vi "UDPTeste.vi"(11 "UDP RX":T1={"Port:"=10020, "Server IP:"="224.5.23.2", "Local IP:"="224.5.23.2", "RX"=FALSE}) -> (2 "RX":bool, 3 "data camera":u8[](array[numeric]))   [LabVIEW 2018]
uses:
  Control/SSL UDP Address.ctl
  <vilib>/Utility/tcp.llb/UDP Multicast Read-Only Open.vi
panel:
  out "error out":errorcluster
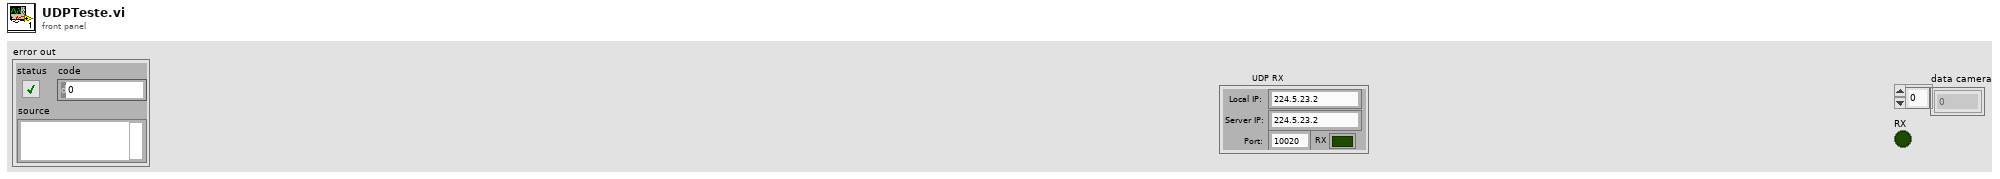
[diagram p1: front panel]
types:
  T1 = typedef "SSL UDP Address.ctl" = cluster{"Port:":u16, "Server IP:":string, "Local IP:":string, "RX":bool}
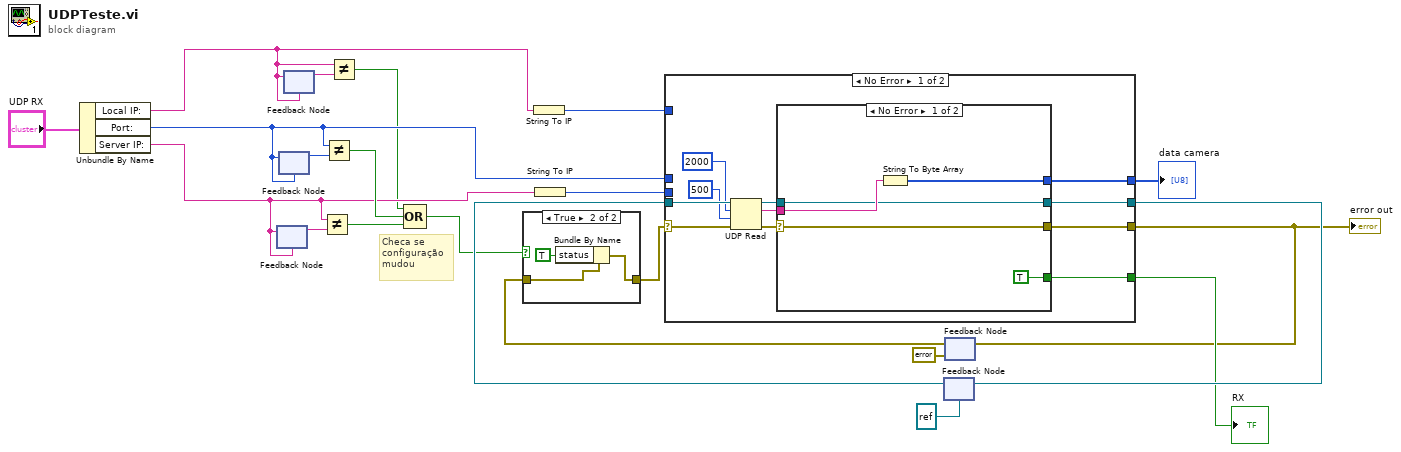
[diagram p0: block diagram]
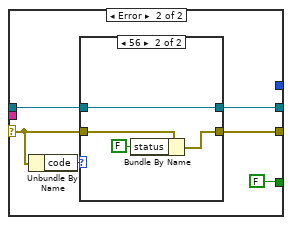
[diagram p3: hidden frame]
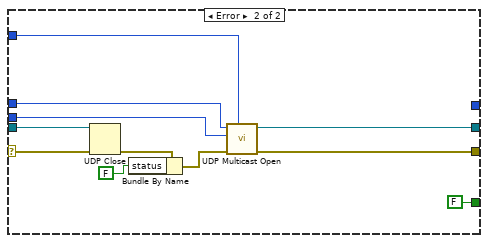
[diagram p5: hidden frame]
diagram:
  # "Checa se \nconfiguração\nmudou"
  n1 = Unbundle By Name("UDP RX") -> ("Local IP:"=w6:string, "Port:"=w10:u16, "Server IP:"=w9:string)
  n2 = feedback #1(w9) -> (w15:string)
  n3 = feedback-in #1(w9) -> ()
  n4 = feedback #2(w10) -> (w13:u16)
  n5 = feedback-in #2(w10) -> ()
  n6 = feedback #3(w6) -> (w8:string)
  n7 = feedback-in #3(w6) -> ()
  n8 = Not Equal?(x=w9, y=w15) -> (x != y?=w14:bool)
  n9 = Not Equal?(x=w10, y=w13) -> (x != y?=w12:bool)
  n10 = Not Equal?(x=w6, y=w8) -> (x != y?=w7:bool)
  n11 = Compound Arithmetic op=OR(w7, w12, w14) -> (w11:bool)
  n12 = String To IP(1:w6) -> (0:w5:u32)
  n13 = String To IP(1:w9) -> (0:w20:u32)
  n14 = feedback #4(refnum<k16> refnum ("connection ID")) -> (w21:refnum<k16>)
  n15 = feedback #5(errorcluster {"status"=TRUE, "code"=0, "source"=""} ("error out")) -> (w17:errorcluster)
  n16 = case shown="True" w11 {
    tunnel: w17 -> [w23 w25]
    tunnel: [w23 w24] -> w16
    frame False {
    }
    frame True {
      n17 = Bundle By Name(cluster=w25, "status"=TRUE) -> (w24:errorcluster)
    }
  }
  n18 = case shown="No Error" w16 {
    selector: w16 -> [w28 w56]
    tunnel: w21 -> [w37 w62]
    tunnel: [w36 w64] -> w3
    tunnel: [w35 w65] -> w22
    tunnel: w10 -> [_ w63]
    tunnel: w20 -> [_ w61]
    tunnel: [w29 FALSE] -> w4
    tunnel: w5 -> [_ w55]
    tunnel: [w27 _] -> w2
    frame No Error {
      n19 = UDP Read(connection ID=w37, max size (548)=2000, timeout ms (25000)=500, 8:w28) -> (data out=w32:string, error out=w30:errorcluster, 3:w31:refnum<k16>)  [unwired: 2 out]
      n20 = case shown="No Error" w30 {
        selector: w30 -> [w39 w43]
        tunnel: w32 -> [w42 _]
        tunnel: [w39 w45] -> w36
        tunnel: [w41 w46] -> w35
        tunnel: w31 -> [w41 w47]
        tunnel: [TRUE FALSE] -> w29
        tunnel: [w38 _] -> w27
        frame No Error {
          n21 = String To Byte Array(string=w42) -> (unsigned byte array=w38:u8[])
        }
        frame Error {
          n22 = Unbundle By Name(w43) -> ("code"=w48:i32)
          n23 = case shown="56" w48 {
            tunnel: w43 -> [w50 w54]
            tunnel: [w50 w52] -> w45
            tunnel: w47 -> [w49 w51]
            tunnel: [w49 w51] -> w46
            frame Default {
            }
            frame 56 {
              n24 = Bundle By Name(cluster=w54, "status"=FALSE) -> (w52:errorcluster)
            }
          }
        }
      }
    }
    frame Error {
      n25 = UDP Close(connection ID=w62, 8:w56) -> (error out=w59:errorcluster)  [unwired: 1 out]
      n26 = Bundle By Name(cluster=w59, "status"=FALSE) -> (w57:errorcluster)
      n27 = call-poly <vilib>:"UDP Multicast Open.vi"("net address"=w55, "error in (no error)"=w57, "multicast addr"=w61, "port"=w63) -> ("error out"=w64:errorcluster, "connection ID"=w65:refnum<k16>)  [unwired: 5 in, 1 out]
    }
  }
  "error out" <- w3
  "data camera" <- w2
  "RX" <- w4
  n28 = feedback-in #4(w22) -> ()
  n29 = feedback-in #5(w3) -> ()
